vi "MeanTempGlobalVar.vi"(8 "Temp In":sgl, 11 "State":enum16{"Initialise", "Write", "Read"}(ring)) -> (3 "Temp out":sgl)   [LabVIEW 2014]
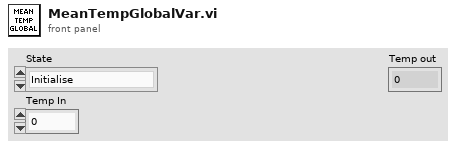
[diagram p1: front panel]
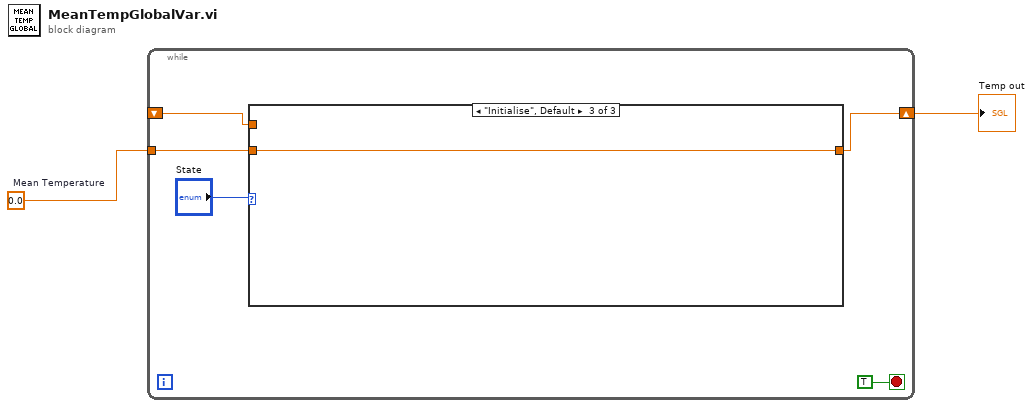
[diagram p0: block diagram]
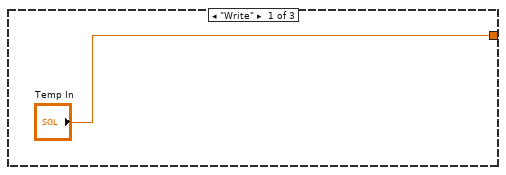
[diagram p2: hidden frame]
diagram:
  w2 = sgl 0.0  # Mean Temperature
  n1 = while {
    tunnel: w2 -> [w5]
    shift-right: [w4] -> w1
    shift-left: _ -> [w3]
    stop <- TRUE stop-if-true
    n2 = case shown="\"Initialise\", Default" "State" {
      tunnel: w5 -> [_ _ w10]
      tunnel: ["Temp In" w9 w10] -> w4
      tunnel: w3 -> [_ w9 _]
      frame "Write" {
      }
      frame "Read" {
      }
      frame "Initialise", Default {
      }
    }
  }
  "Temp out" <- w1
